vi "Test_IncrementValuePublication_String_ErrorReturned.vi"(8 "error in (no error)":errorcluster, 11 "TestCase in":refnum<class "TestPublicationPolicy.lvclass">) -> (0 "error out":errorcluster, 3 "TestCase out":refnum<class "TestPublicationPolicy.lvclass">)   [LabVIEW 2020, in "TestPublicationPolicy.lvclass"]
uses:
  TestPublicationPolicy.lvclass
  TestPublicationPolicy.lvclass/TestPublicationPolicy.ctl
  Source/PublicationPolicy/IncrementValuePublication/IncrementValuePublication.lvclass
  Source/IMediator/MutexedPublishRequest/MutexedPublishRequest.lvclass
  Source/IMediator/IPublicationPolicy/IPublicationPolicy.lvclass
  modules/composed-transport/Source/Concrete/NotifierTransport/NotifierTransport.lvclass
  C:/Git/mva-core/Source/IMediator/IPublicationPolicy/IPublicationPolicy.lvclass
  C:/Git/mva-core/Source/PublicationPolicy/IncrementValuePublication/IncrementValuePublication.lvclass
  C:/Git/mva-core/modules/composed-transport/Source/ITransport/ITransport.lvclass
  C:/Git/mva-core/modules/composed-transport/Source/Concrete/NotifierTransport/NotifierTransport.lvclass
panel:
  out "Publish Return Error":errorcluster
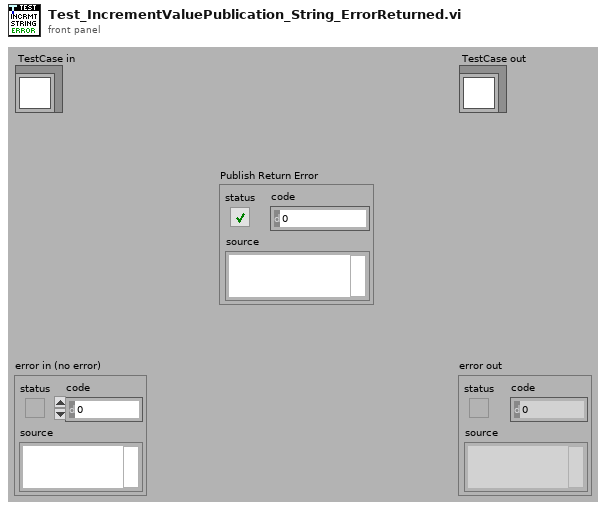
[diagram p1: front panel]
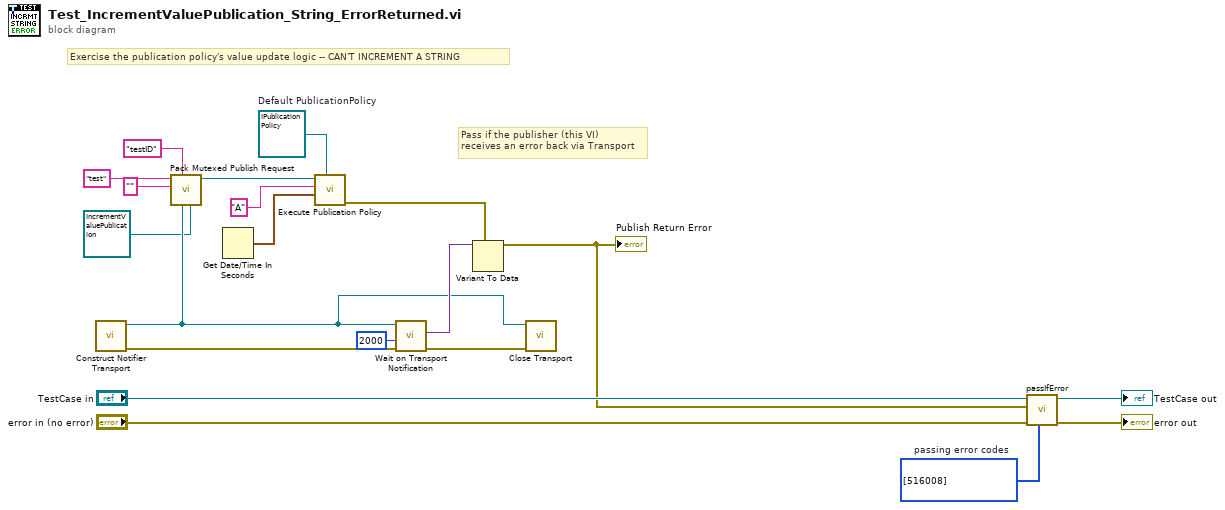
[diagram p0: block diagram]
diagram:
  w4 = i32[] [516008]  # passing error codes
  w13 = refnum<class "IPublicationPolicy.lvclass"> refnum  # Default PublicationPolicy
  # "Pass if the publisher (this VI)\nreceives an error back via Transport"
  # "Exercise the publication policy's value update logic -- CAN'T INCREMENT A STRING"
  n1 = call "Construct Notifier Transport.vi"() -> ("error out"=w9:errorcluster, "NotifierTransport"=w3:refnum<class "NotifierTransport.lvclass">)  [unwired: 10 in]
  n2 = call "Pack Mutexed Publish Request.vi"("PublicationPolicy"=refnum<class "IncrementValuePublication.lvclass"> refnum ("PublicationPolicy.lvlib:IncrementValuePublication.lvclass"), "Return Error Transport"=w3, "Publisher ID"="testID", "Datum Value or Type"="" ("Data to Publish"), "Datum Name"="test") -> ("MutexedPublishRequest Out"=w14:refnum<class "MutexedPublishRequest.lvclass">)  [unwired: 5 in, 1 out]
  n3 = Get Date/Time In Seconds() -> (seconds since 1Jan1904=w15:timestamp)
  n4 = call-dynamic "Execute Publication Policy.vi"("Default PublicationPolicy"=w13, "Last Publish Time"=w15, "Last Published Value"="A", "MutexedPublishRequest"=w14) -> ("error out (Reject Publication)"=w6:errorcluster)  [unwired: 5 in, 2 out]
  n5 = call "Wait on Transport Notification.vi"("error in (no error)"=w9, "Timeout In ms (-1)"=2000, "NotifierTransport"=w3) -> ("error out"=w2:errorcluster, "Data"=w7:variant)  [unwired: 6 in, 1 out]
  n6 = Variant To Data(type=w6, Variant=w7) -> (data=w5:errorcluster)  [unwired: 1 in, 1 out]
  "Publish Return Error" <- w5
  n7 = call-dynamic "Close Transport.vi"("error in (no error)"=w2, "NotifierTransport"=w3) -> ()  [unwired: 9 in, 1 out]
  n8 = call-dynamic "passIfError.vi"("passing error codes (default = any error code)"=w4, "error in (no error)"="error in (no error)", "error"=w5, "TestCase in"="TestCase in") -> ("error out"=→"error out":errorcluster, "TestCase out"=→"TestCase out":refnum<class "TestPublicationPolicy.lvclass">)  [unwired: 6 in]
